vi "Read Message Screen.vi"(8 "error in (no error)":errorcluster, 11 "Simulated Display Console Actor in":refnum<class "Simulated Display Console Actor.lvclass">) -> (0 "error out":errorcluster, 2 "Message Screen":refnum<vi>, 3 "Simulated Display Console Actor out":refnum<class "Simulated Display Console Actor.lvclass">)   [LabVIEW 2019, in "Simulated Display Console Actor.lvlib" / "Simulated Display Console Actor.lvclass"]
uses:
  Simulated Display Console Actor.lvclass
  Simulated Display Console Actor.lvclass/Simulated Display Console Actor.ctl
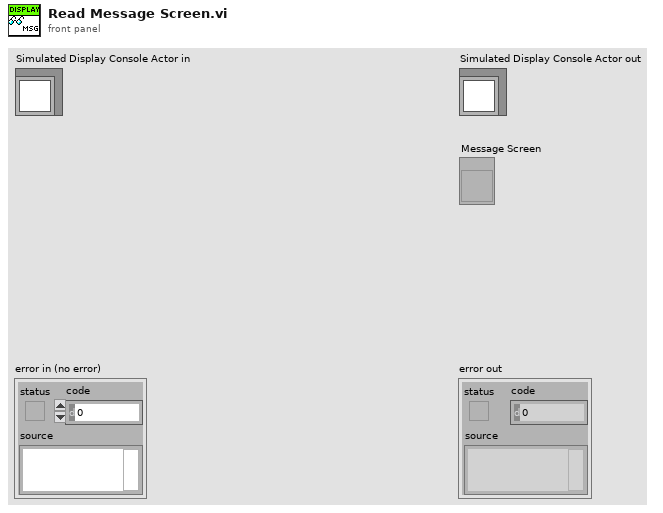
[diagram p1: front panel]
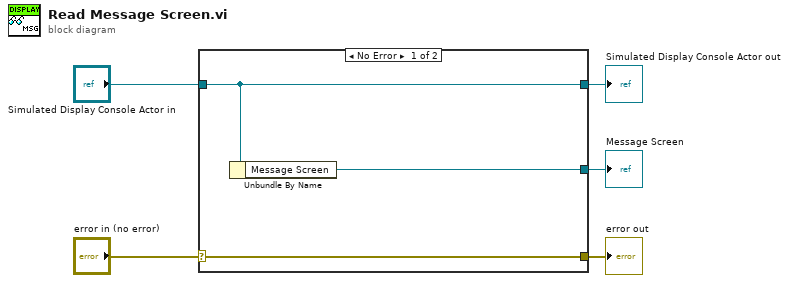
[diagram p0: block diagram]
diagram:
  n1 = case shown="No Error" "error in (no error)" {
    selector: "error in (no error)" -> [w8 w9]
    tunnel: [w8 w9] -> w4
    tunnel: [w7 w10] -> w2
    tunnel: "Simulated Display Console Actor in" -> [w7 w10]
    tunnel: [w6 _] -> w1
    frame No Error {
      n2 = Unbundle By Name(w7) -> ("Message Screen"=w6:refnum<vi>)
    }
    frame Error {
    }
  }
  "error out" <- w4
  "Simulated Display Console Actor out" <- w2
  "Message Screen" <- w1
